vi "(BASVR) Choose Channel & Excitation.vi"(8 "Channel Legend & Control":string[][](array[string]), 9 "Channel Start TIme":timestamp, 10 "Channel Override":u16, 11 "Expected Channel Index":i32) -> (0 "Channel Changed?":bool, 1 "Chosen Excitaiton":u8, 2 "Chosen Channel":i32, 3 "Chosen Channel Index":i32)   [LabVIEW 2023]
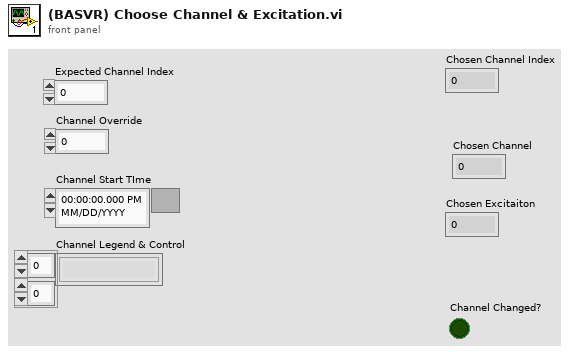
[diagram p1: front panel]
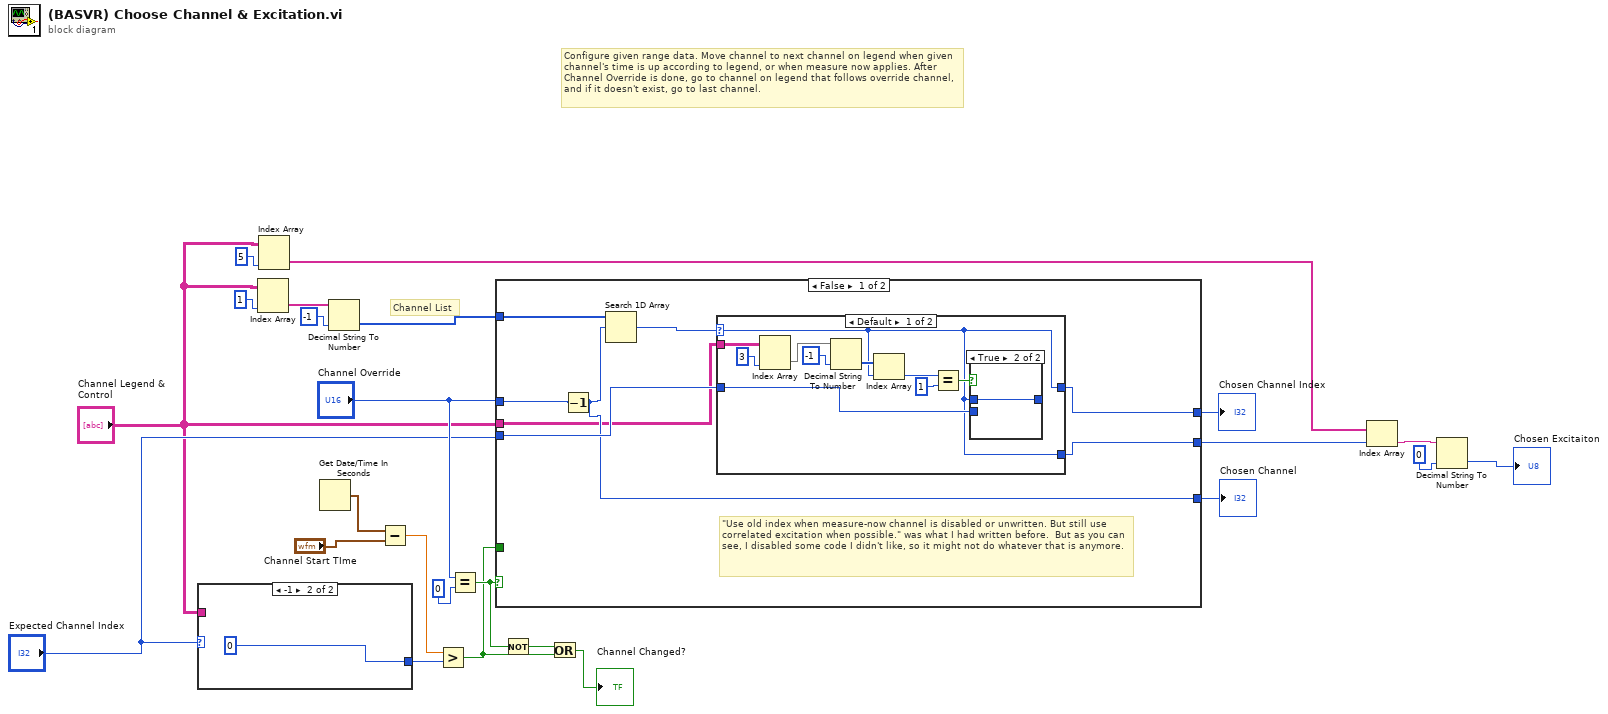
[diagram p0: block diagram]
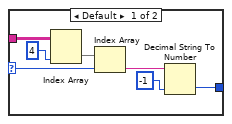
[diagram p2: hidden frame]
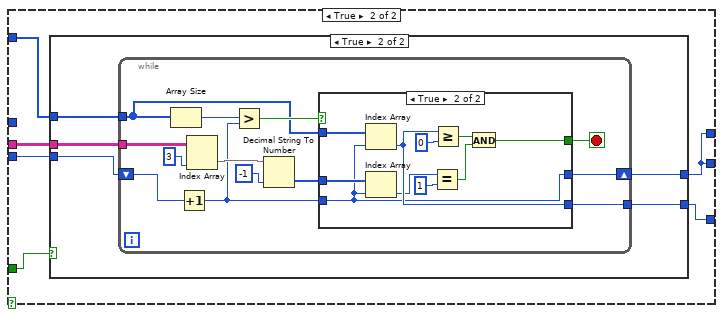
[diagram p5: hidden frame]
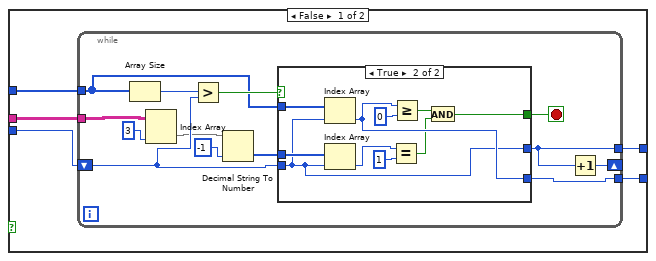
[diagram p6: hidden frame]
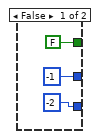
[diagram p7: hidden frame]
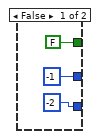
[diagram p8: hidden frame]
diagram:
  # "Channel List"
  # "Configure given range data. Move channel to next channel on legend when given channel's time is up according to legend, or when measure now applies. After Channel Override is done, go to channel on legend that follows override channel, and if it doesn't exist, go to last channel."
  n1 = case shown="-1" "Expected Channel Index" {
    selector: "Expected Channel Index" -> [w26 _]
    tunnel: "Channel Legend & Control" -> [w27 _]
    tunnel: [w25 0] -> w6
    frame Default {
      n2 = Index Array(array=w27, index (col)=4 ("index (row)")) -> (element=w30:string[])  [unwired: 1 in]
      n3 = Index Array(array=w30, index=w26) -> (element=w31:string)
      n4 = Decimal String To Number(string=w31, default (0L)=-1 ("default (0 I32)")) -> (number=w25:i32)  [unwired: 1 in, 1 out]
    }
    frame -1 {
    }
  }
  n5 = Index Array(array="Channel Legend & Control", index (col)=1 ("index (row)")) -> (element=w22:string[])  [unwired: 1 in]
  n6 = Index Array(array="Channel Legend & Control", index (col)=5 ("index (row)")) -> (element=w18:string[])  [unwired: 1 in]
  n7 = Get Date/Time In Seconds() -> (seconds since 1Jan1904=w3:timestamp)
  n8 = Decimal String To Number(string=w22, default (0L)=-1 ("default (0 I32)")) -> (number=w20:i32[])  [unwired: 1 in, 1 out]
  n9 = Subtract(x=w3, y="Channel Start TIme") -> (x-y=w24:dbl)
  n10 = Greater?(x=w24, y=w6) -> (0:w5:bool)
  n11 = Equal?(x="Channel Override", y=u16 0) -> (x = y?=w9:bool)
  n12 = case shown="False" w9 {
    tunnel: "Expected Channel Index" -> [w39 w59]
    tunnel: w5 -> [_ w58]
    tunnel: [w36 w57] -> w23
    tunnel: [w38 w54] -> w17
    tunnel: "Channel Override" -> [w37 _]
    tunnel: w20 -> [w40 w56]
    tunnel: "Channel Legend & Control" -> [w35 w55]
    tunnel: [w33 w54] -> w1
    frame False {
      # "\"Use old index when measure-now channel is disabled or unwritten. But still use correlated excitation when possible.\" was what I had written before.  But as you can see, I disabled some code I didn't like, so it might not do whatever that is anymore."
      n13 = Decrement(x=w37) -> (x-1=w36:u16)
      n14 = Search 1D Array(1D array=w40, element=w36) -> (index of element=w34:i32)  [unwired: 1 in]
      n15 = case shown="Default" w34 {
        selector: w34 -> [w41 _]
        tunnel: w39 -> [w42 w53]
        tunnel: [w41 w53] -> w38
        tunnel: w35 -> [w47 _]
        tunnel: [w41 w53] -> w33
        frame Default {
          n16 = Index Array(array=w47, index (col)=3 ("index (row)")) -> (element=w49:string[])  [unwired: 1 in]
          n17 = Decimal String To Number(string=w49, default (0L)=-1 ("default (0 I32)")) -> (number=w50:i32[])  [unwired: 1 in, 1 out]
          n18 = Index Array(array=w50, index=w41) -> (element=w44:i32)
          n19 = Equal?(x=w44, y=1) -> (x = y?=w43:bool)
          n20 = case shown="True" w43 {
            tunnel: w42 -> [w51 _]
            tunnel: w41 -> [_ w52]
            tunnel: [w51 w52] -> _
            frame False {
            }
            frame True {
            }
          }
        }
        frame -1 {
        }
      }
    }
    frame True {
      n21 = case shown="True" w58 {
        tunnel: w59 -> [w62 w91]
        tunnel: [w63 w92] -> w57
        tunnel: [w61 w93] -> w54
        tunnel: w56 -> [w64 w95]
        tunnel: w55 -> [w60 w94]
        frame False {
          n22 = while {
            shift-right: [w71] -> _
            shift-left: w62 -> [w72]
            tunnel: [w74] -> w63
            tunnel: w64 -> [w73]
            tunnel: [w70] -> w61
            tunnel: w60 -> [w67]
            stop <- w77 stop-if-true
            n23 = Array Size(array=w73) -> (size(s)=w76:i32)
            n24 = Index Array(array=w67, index (col)=3 ("index (row)")) -> (element=w69:string[])  [unwired: 1 in]
            n25 = Greater?(x=w76, y=w72) -> (0:w75:bool)
            n26 = Decimal String To Number(string=w69, default (0L)=-1 ("default (0 I32)")) -> (number=w66:i32[])  [unwired: 1 in, 1 out]
            n27 = case shown="True" w75 {
              tunnel: w72 -> [_ w81]
              tunnel: w73 -> [_ w90]
              tunnel: [FALSE w83] -> w77
              tunnel: [-1 w81] -> w70
              tunnel: [-2 w88] -> w74
              tunnel: w66 -> [_ w87]
              frame False {
              }
              frame True {
                n28 = Index Array(array=w90, index=w81) -> (element=w88:i32)
                n29 = Index Array(array=w87, index=w81) -> (element=w86:i32)
                n30 = Equal?(x=w86, y=1) -> (x = y?=w82:bool)
                n31 = Greater Or Equal?(x=w88, y=0) -> (x >= y?=w84:bool)
                n32 = And(x=w84, y=w82) -> (x .and. y?=w83:bool)
              }
            }
            n33 = Increment(x=w70) -> (x+1=w71:i32)
          }
        }
        frame True {
          n34 = while {
            tunnel: w95 -> [w102]
            tunnel: w94 -> [w101]
            tunnel: [w98] -> w92
            shift-right: [w99] -> w93
            shift-left: w91 -> [w96]
            stop <- w97 stop-if-true
            n35 = Array Size(array=w102) -> (size(s)=w108:i32)
            n36 = Increment(x=w96) -> (x+1=w100:i32)
            n37 = Index Array(array=w101, index (col)=3 ("index (row)")) -> (element=w106:string[])  [unwired: 1 in]
            n38 = Greater?(x=w108, y=w100) -> (0:w107:bool)
            n39 = Decimal String To Number(string=w106, default (0L)=-1 ("default (0 I32)")) -> (number=w104:i32[])  [unwired: 1 in, 1 out]
            n40 = case shown="True" w107 {
              tunnel: w100 -> [_ w112]
              tunnel: w102 -> [_ w121]
              tunnel: [FALSE w114] -> w97
              tunnel: [-1 w112] -> w99
              tunnel: [-2 w119] -> w98
              tunnel: w104 -> [_ w118]
              frame False {
              }
              frame True {
                n41 = Index Array(array=w121, index=w112) -> (element=w119:i32)
                n42 = Index Array(array=w118, index=w112) -> (element=w117:i32)
                n43 = Equal?(x=w117, y=1) -> (x = y?=w113:bool)
                n44 = Greater Or Equal?(x=w119, y=0) -> (x >= y?=w115:bool)
                n45 = And(x=w115, y=w113) -> (x .and. y?=w114:bool)
              }
            }
          }
        }
      }
    }
  }
  "Chosen Channel" <- w23
  "Chosen Channel Index" <- w17
  n46 = Not(x=w9) -> (.not. x?=w2:bool)
  n47 = Or(x=w2, y=w5) -> (x .or. y?=→"Channel Changed?":bool)
  n48 = Index Array(array=w18, index=w1) -> (element=w16:string)
  n49 = Decimal String To Number(string=w16, default (0L)=0 ("default (0 I32)")) -> (number=→"Chosen Excitaiton":i32)  [unwired: 1 in, 1 out]
